vi "AFT Filter Signal and Update Coefficients (Complex, Array).vi"(6 "step size":dbl=-1.0, 7 "reset? (F)":bool, 8 "error in (no error)":errorcluster, 9 "d(n)":cdb[](array[numeric]), 10 "x(n)":cdb[](array[numeric]), 11 "adaptive filter in":refnum<k20>) -> (0 "error out":errorcluster, 1 "e(n)":cdb[](array[numeric]), 2 "y(n)":cdb[](array[numeric]), 3 "adaptive filter out":refnum<k20>)   [LabVIEW 2017, in "NI_AdaptiveFilter.lvlib"]
doc: "Filters an input signal with an adaptive filter and updates the coefficients of the adaptive filter iteratively. You must use the least mean squares (LMS) or recursive least squares (RLS) algorithms to create the adaptive filter. Wire data to the <B>x(n)</B> and <B>d(n)</B> inputs to determine the polymorphic instance to use or manually select the instance. The data type of the adaptive filter that you wire to the <B>adaptive filter in</B> input must match the instance of the AFT Filter Signal and Update Coefficients VI."
uses:
  <vilib>/addons/Adaptive Filters/NI_AdaptiveFilter.lvlib
  <resource>/AdaptiveFilters.dll
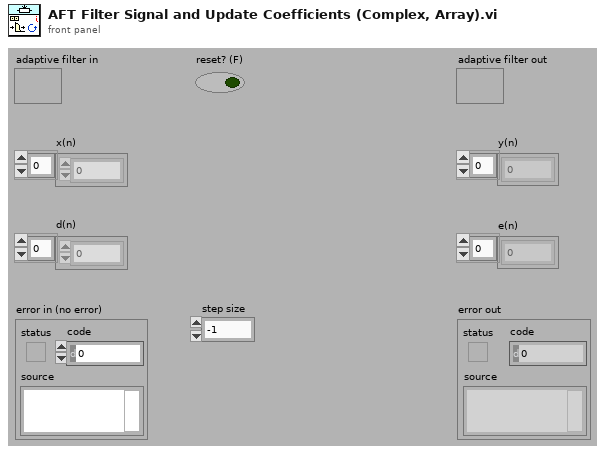
[diagram p1: front panel]
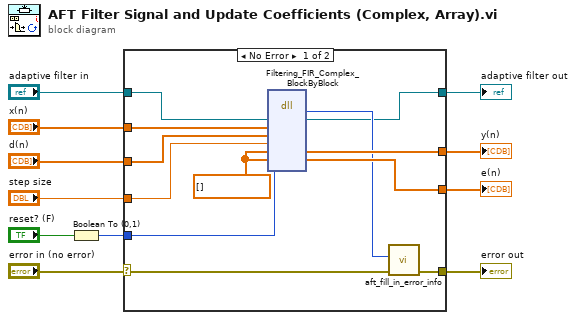
[diagram p0: block diagram]
diagram:
  n1 = Boolean To (0,1)(Boolean="reset? (F)") -> (0, 1=w9:i16)
  n2 = case shown="No Error" "error in (no error)" {
    selector: "error in (no error)" -> [w19 w25]
    tunnel: [w17 w25] -> w11
    tunnel: "adaptive filter in" -> [w13 w24]
    tunnel: "x(n)" -> [w23 _]
    tunnel: "d(n)" -> [w22 _]
    tunnel: [w21 _] -> w3
    tunnel: [w20 _] -> w2
    tunnel: [w12 w24] -> w7
    tunnel: w9 -> [w16 _]
    tunnel: "step size" -> [w15 _]
    frame No Error {
      w14 = cdb[] [] ("d(n)")
      n3 = dll-call lib="C:/Program Files/National Instruments/LabVIEW 2017/resource/AdaptiveFilters.dll" fn="Filtering_FIR_Complex_BlockByBlock"("pSession"=w13, "x"=w23, "d"=w22, "mu"=w15, "y"=w14, "e"=w14, "reset"=w16) -> ("err"=w18:i32, "pSession"=w12:refnum<k20>, "y"=w21:cdb[], "e"=w20:cdb[])  [unwired: 7 in, 2 out]
      n4 = call <vilib>:"aft_fill_in_error_info.vi"("error in"=w19, "status code"=w18) -> ("error out"=w17:errorcluster)  [unwired: 2 in, 7 out]
    }
    frame Error {
    }
  }
  "error out" <- w11
  "adaptive filter out" <- w7
  "y(n)" <- w3
  "e(n)" <- w2
